vi "VoltageTest.vi"() -> ()   [LabVIEW 2019]
uses:
  <instrlib>/niDMM/nidmm.llb/niDMM Function.ctl
  <instrlib>/niDMM/nidmm.llb/niDMM Resolution in Digits.ctl
  <instrlib>/niDMM/nidmm.llb/niDMM Configure Measurement Digits.vi
panel:
  in  "Instrument Descriptor":refnum<k15>
  in  "Self-Calibrate at the beginning?":bool
  in  "Range (Volts)":dbl=10.0 format="%.2p"
  out "Waveform Chart":dbl(graph)
  out "Over Range?":bool
  out "Measurement (Volts)":dbl format="%_7p"
  in  "Resolution in Digits":T1=5.5 items=["3 1/2"=3.5, "4 1/2"=4.5, "5 1/2"=5.5, "6 1/2"=6.5, "7 1/2"=7.5]
  in  "Function":T2
  in  "stop":bool
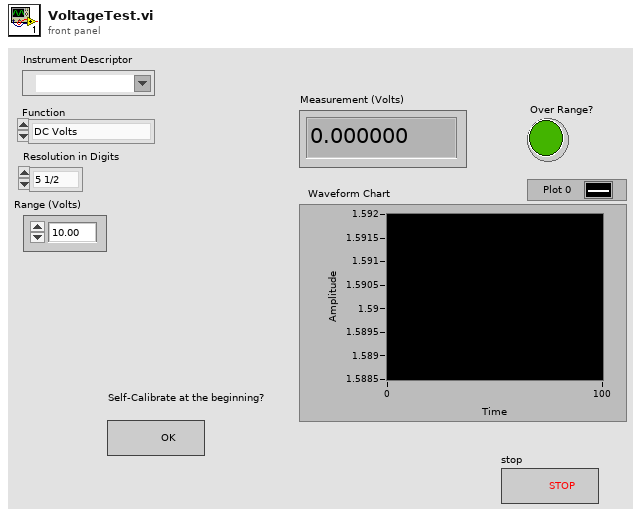
[diagram p1: front panel]
types:
  T1 = typedef "niDMM Resolution in Digits.ctl" = dbl
  T2 = typedef "niDMM Function.ctl" = enum16{"DC Volts", "AC Volts", "DC Current", "AC Current", "2-wire Resistance", "4-wire Resistance", "Diode", "Frequency", "Period", "AC Volts DC Coupled", "Capacitance", "Inductance", "Temperature"}
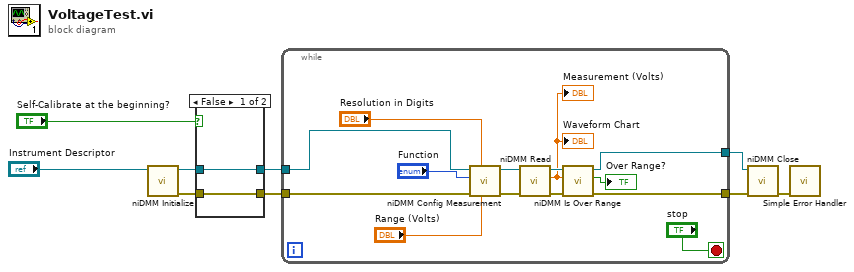
[diagram p0: block diagram]
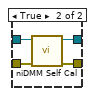
[diagram p2: hidden frame]
diagram:
  n1 = call <instrlib>:"niDMM Initialize.vi"("Instrument Descriptor"="Instrument Descriptor") -> ("error out"=w4:errorcluster, "instrument handle out"=w5:refnum<k15>)  [unwired: 9 in]
  n2 = case shown="False" "Self-Calibrate at the beginning?" {
    tunnel: w5 -> [w11 w15]
    tunnel: w4 -> [w10 w14]
    tunnel: [w10 w13] -> w1
    tunnel: [w11 w12] -> w2
    frame False {
    }
    frame True {
      n3 = call <instrlib>:"niDMM Self Cal.vi"("error in (no error)"=w14, "instrument handle"=w15) -> ("error out"=w13:errorcluster, "instrument handle out"=w12:refnum<k15>)  [unwired: 8 in]
    }
  }
  n4 = while {
    tunnel: [w22] -> w8
    tunnel: [w21] -> w7
    tunnel: w2 -> [w17]
    tunnel: w1 -> [w16]
    stop <- "stop" stop-if-true
    n5 = call-poly <instrlib>:"niDMM Config Measurement.vi"("Range"="Range (Volts)", "Resolution in Digits"="Resolution in Digits", "error in (no error)"=w16, "Function"="Function", "instrument handle"=w17) -> ("error out"=w25:errorcluster, "instrument handle out"=w26:refnum<k15>)  [unwired: 5 in]
    n6 = call <instrlib>:"niDMM Read.vi"("error in (no error)"=w25, "instrument handle"=w26) -> ("error out"=w23:errorcluster, "Measurement"=w19:dbl, "instrument handle out"=w24:refnum<k15>)  [unwired: 7 in]
    "Measurement (Volts)" <- w19
    "Waveform Chart" <- w19
    n7 = call <instrlib>:"niDMM Is Over Range.vi"("error in (no error)"=w23, "Measurement"=w19, "instrument handle"=w24) -> ("error out"=w21:errorcluster, "Over Range?"=→"Over Range?":bool, "instrument handle out"=w22:refnum<k15>)  [unwired: 6 in]
  }
  n8 = call <instrlib>:"niDMM Close.vi"("error in (no error)"=w7, "instrument handle"=w8) -> ("error out"=w9:errorcluster)  [unwired: 9 in]
  n9 = call <vilib>:"Simple Error Handler.vi"("error in (no error)"=w9) -> ()  [unwired: 4 in, 5 out]
